vi "GetParam.vi"(8 "error in (no error)":errorcluster caption="entrée d'erreur (pas d'erreur)", 11 "Rbf_kernel.lvclass":refnum<class "Rbf_kernel.lvclass">) -> (0 "error out":errorcluster caption="sortie d'erreur", 2 "rbf_kernel":cluster{"gamma":string}={"gamma"="None"}, 3 "Rbf_kernel.lvclass":refnum<class "Rbf_kernel.lvclass">)   [LabVIEW 2020, in "Rbf_kernel.lvclass"]
doc: "Get Parameters"
uses:
  Rbf_kernel.lvclass
  Rbf_kernel.lvclass/Rbf_kernel.ctl
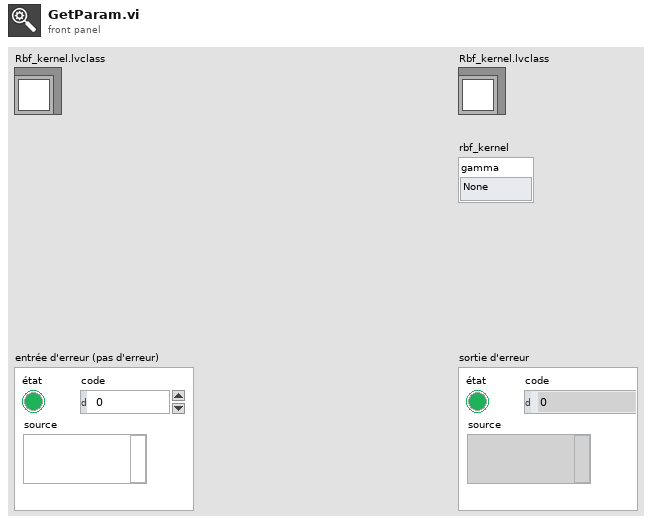
[diagram p1: front panel]
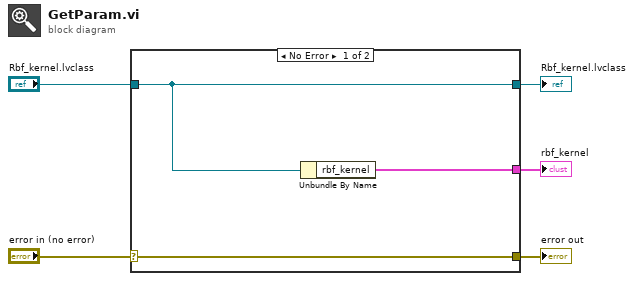
[diagram p0: block diagram]
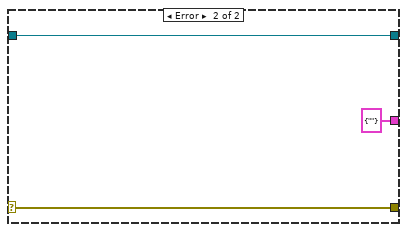
[diagram p2: hidden frame]
diagram:
  n1 = case shown="No Error" "error in (no error)" {
    selector: "error in (no error)" -> [w8 w10]
    tunnel: [w8 w10] -> w4
    tunnel: [w7 w11] -> w2
    tunnel: "Rbf_kernel.lvclass" -> [w7 w11]
    tunnel: [w6 cluster{"gamma":string} {"gamma"=""} ("rbf_kernel")] -> w1
    frame No Error {
      n2 = Unbundle By Name(w7) -> ("rbf_kernel"=w6:cluster{"gamma":string})
    }
    frame Error {
    }
  }
  "error out" <- w4
  "Rbf_kernel.lvclass" <- w2
  "rbf_kernel" <- w1
